vi "FlexRIOonlyResources.vi"() -> ()   [LabVIEW 2013]
uses:
  Control 1.ctl
  ctl.ctl
  <vilib>/Platform/TimedLoop/XDataNode/timing_clust.ctl
  <vilib>/Platform/TimedLoop/XDataNode/nitl_modes.ctl
  <vilib>/Platform/TimedLoop/XDataNode/wakeup.ctl
  Libraries/StateControl.ctl
  Libraries/FlexRIO-NoModule/N Channels.ctl
  <vilib>/rvi/Emulation/niFpgaSctlEmulationGetInTimedLoop.vi
  <vilib>/rvi/Emulation/niFpgaEmulationReportErrorSimple.vi
  <vilib>/rvi/Emulation/niFpgaGetClockAttributes.vi
  <vilib>/rvi/Emulation/niFpgaCriticalErrorInLSC.vi
  <vilib>/rvi/FIFO/Fifo_Resource/nirvififoEmulationClearFpgaImpl.vi
  <vilib>/rvi/DataTransferAndStorage/Container/Common/niFpgaContainerGetUniqueNameForEmu.vi
  Libraries/GlobalReg.vi
  <vilib>/rvi/DataTransferAndStorage/Container/Common/niFpgaContainerExecOnDevCompGetState.vi
  <vilib>/rvi/FIFO/Fifo_Resource/nirvififoEmulationGetNumberOfElementsToReadFpgaImpl.vi
  <vilib>/rvi/interface/RandomDataEmulation/nirviRandomDataFPGAFIFO.vi
  <vilib>/rvi/interface/RandomDataEmulation/niFpgaRandomDataHandleErrors.vi
  <vilib>/rvi/eio/common/nirviEmuReportErrorAndStop.vi
  <vilib>/rvi/FIFO/Fifo_Resource/nirvififoEmulationReadFpgaImpl.vi
  <vilib>/rvi/FIFO/Fifo_Resource/nirvififoEmulationWriteFpgaImpl.vi
  <vilib>/rvi/Emulation/niFpgaProcessEmulError.vi
  <vilib>/rvi/eio/common/nirviEmuTemplateMethod_errors.vi
  <vilib>/Platform/TimedLoop/XDataNode/XDataNode.xnode
  <vilib>/rvi/DataTransferAndStorage/Container/XNode/niFpgaContainer.xnode
  <vilib>/rvi/FIFO/Fifo_Resource/nirvififoEmulationClear.vi
  <vilib>/rvi/FIFO/Fifo_Resource/niFpgaFifoEmulationRefIn.vi
  <vilib>/rvi/interface/RandomDataEmulation/nirviRandomDataFpgaReadWriteTemplate.vi
  <vilib>/eio/EIONode/EIONode.xnode
  <vilib>/Platform/TimedLoop/XDataNode/XDNodeRunTimeDep.lvlib
panel:
  in  "Cluster in":T1
  in  "Tab Control":T2(tab)=enum."Data Acquisition"
  out "Platform":enum8{"FlexRIO", "cRIO", "RSeries"}(ring)
  out "FPGAVIversion":u8[](array[numeric])=[1, 1]
  out "InitDone":bool
  out "RIOAdapterCorrect":bool
  out "Fref":u32=100000000
  out "DevQualityStatus":u8
  out "DevTemp":i16=-10244
  out "DevProfile":u8 format="%x"
  in  "DAQStartStop":bool
  in  "DebugMode":bool
  out "Expected IO Module ID":u32 format="%x"
  out "InsertedIOModule ID":u32
  out "DMATtoHOSTNCh":T3[](array[typedef])=[4]
  out "DMATtoHOSTFrameType":u8[](array[numeric])
  out "DMATtoHOSTSampleSize":u8[](array[numeric])=[2]
  out "DMATtoHOSTBlockNWords":u16[](array[numeric])=[4096]
  in  "DMATtoHOSTSamplingRate0":u16=10000
  in  "DMATtoHOSTEnable0":bool
  out "DMATtoHOSTOverflows":u16
  out "auxAI5":i32
  out "auxAI4":i32
  out "auxAI3":i32
  out "auxAI2":i32
  out "auxAI1":i32
  out "auxAI0":i32
  in  "auxAO5":i32
  in  "auxAO4":i32
  in  "auxAO3":i32
  in  "auxAO2":i32
  in  "auxAO1":i32
  in  "auxAO0":i32
  out "auxDI5":bool
  out "auxDI4":bool
  out "auxDI3":bool
  out "auxDI2":bool
  out "auxDI1":bool
  out "auxDI0":bool
  in  "auxDO3":bool
  in  "auxDO4":bool
  in  "auxDO5":bool
  in  "auxDO2":bool
  in  "auxDO1":bool
  in  "auxDO0":bool
  in  "AOEnable0":bool
  in  "SGUpdateRate0":u32=40
  in  "SGSignalType0":u8
  in  "SGPhase0":u32
  in  "SGFreq0":u32=100000
  in  "SGAmp0":u16
  in  "AO0":i32
  out "SGNo":u8=2 format="%x"
  out "SGFref0":u32=100000000
  out "auxDI6":bool
  out "auxDI7":bool
  out "auxDI8":bool
  out "auxDI9":bool
  out "auxDI10":bool
  out "auxDI11":bool
  out "auxDI12":bool
  out "auxDI13":bool
  out "auxDI14":bool
  out "auxDI15":bool
  in  "auxDO6":bool
  in  "auxDO7":bool
  in  "auxDO8":bool
  in  "auxDO12":bool
  in  "auxDO13":bool
  in  "auxDO14":bool
  in  "auxDO11":bool
  in  "auxDO10":bool
  in  "auxDO9":bool
  in  "auxDO15":bool
  in  "auxAO6":i32
  in  "auxAO7":i32
  in  "auxAO8":i32
  in  "auxAO9":i32
  in  "auxAO10":i32
  in  "auxAO11":i32
  in  "auxAO12":i32
  in  "auxAO13":i32
  in  "auxAO14":i32
  in  "auxAO15":i32
  out "auxAI6":i32
  out "auxAI7":i32
  out "auxAI8":i32
  out "auxAI9":i32
  out "auxAI10":i32
  out "auxAI11":i32
  out "auxAI12":i32
  out "auxAI13":i32
  out "auxAI14":i32
  out "auxAI15":i32
  in  "AOEnable1":bool
  in  "AO1":i32
  in  "SGUpdateRate1":u32=40
  in  "SGFreq1":u32=100000
  out "SGFref1":u32=100000000
  in  "SGPhase1":u32
  in  "SGAmp1":u16
  in  "SGSignalType1":u8
  in  "DO15":bool
  in  "DO14":bool
  in  "DO13":bool
  in  "DO12":bool
  in  "DO9":bool
  in  "DO10":bool
  in  "DO11":bool
  in  "DO8":bool
  in  "DO7":bool
  in  "DO6":bool
  in  "DO3":bool
  in  "DO4":bool
  in  "DO5":bool
  in  "DO2":bool
  in  "DO1":bool
  in  "DO0":bool
  in  "DO18":bool
  in  "DO19":bool
  in  "DO20":bool
  in  "DO17":bool
  in  "DO16":bool
  in  "DO21":bool
  in  "DO24":bool
  in  "DO25":bool
  in  "DO26":bool
  in  "DO23":bool
  in  "DO22":bool
  in  "DO27":bool
  in  "DO30":bool
  in  "DO31":bool
  in  "DO32":bool
  in  "DO33":bool
  in  "DO36":bool
  in  "DO37":bool
  in  "DO38":bool
  in  "DO29":bool
  in  "DO28":bool
  in  "DO39":bool
  in  "DO42":bool
  in  "DO43":bool
  in  "DO44":bool
  in  "DO35":bool
  in  "DO34":bool
  in  "DO45":bool
  in  "DO48":bool
  in  "DO49":bool
  in  "DO50":bool
  in  "DO51":bool
  in  "DO52":bool
  in  "DO40":bool
  in  "DO41":bool
  in  "DO53":bool
  in  "DO46":bool
  in  "DO47":bool
  out "DI11":bool
  out "DI10":bool
  out "DI9":bool
  out "DI8":bool
  out "DI7":bool
  out "DI6":bool
  out "DI15":bool
  out "DI14":bool
  out "DI13":bool
  out "DI12":bool
  out "DI5":bool
  out "DI4":bool
  out "DI3":bool
  out "DI2":bool
  out "DI1":bool
  out "DI0":bool
  out "DI18":bool
  out "DI19":bool
  out "DI20":bool
  out "DI21":bool
  out "DI22":bool
  out "DI23":bool
  out "DI30":bool
  out "DI31":bool
  out "DI32":bool
  out "DI33":bool
  out "DI24":bool
  out "DI25":bool
  out "DI26":bool
  out "DI27":bool
  out "DI28":bool
  out "DI29":bool
  out "DI36":bool
  out "DI37":bool
  out "DI38":bool
  out "DI39":bool
  out "DI40":bool
  out "DI41":bool
  out "DI34":bool
  out "DI35":bool
  out "DI16":bool
  out "DI17":bool
  out "DI42":bool
  out "DI43":bool
  out "DI44":bool
  out "DI45":bool
  out "DI46":bool
  out "DI47":bool
  out "DI51":bool
  out "DI52":bool
  out "DI53":bool
  out "DI48":bool
  out "DI49":bool
  out "DI50":bool
  # "Inputs"
  # "Aux Analog Input"
  # "Aux Digital Input"
  # "Digital Inputs"
  # "Outputs"
  # "Analog Outputs"
  # "Number of WF gen"
  # "Digital Outputs"
  # "Signal Generator 0"
  # "Signal Generator 1"
  # "Aux Digital Output"
  # "Aux Analog Output"
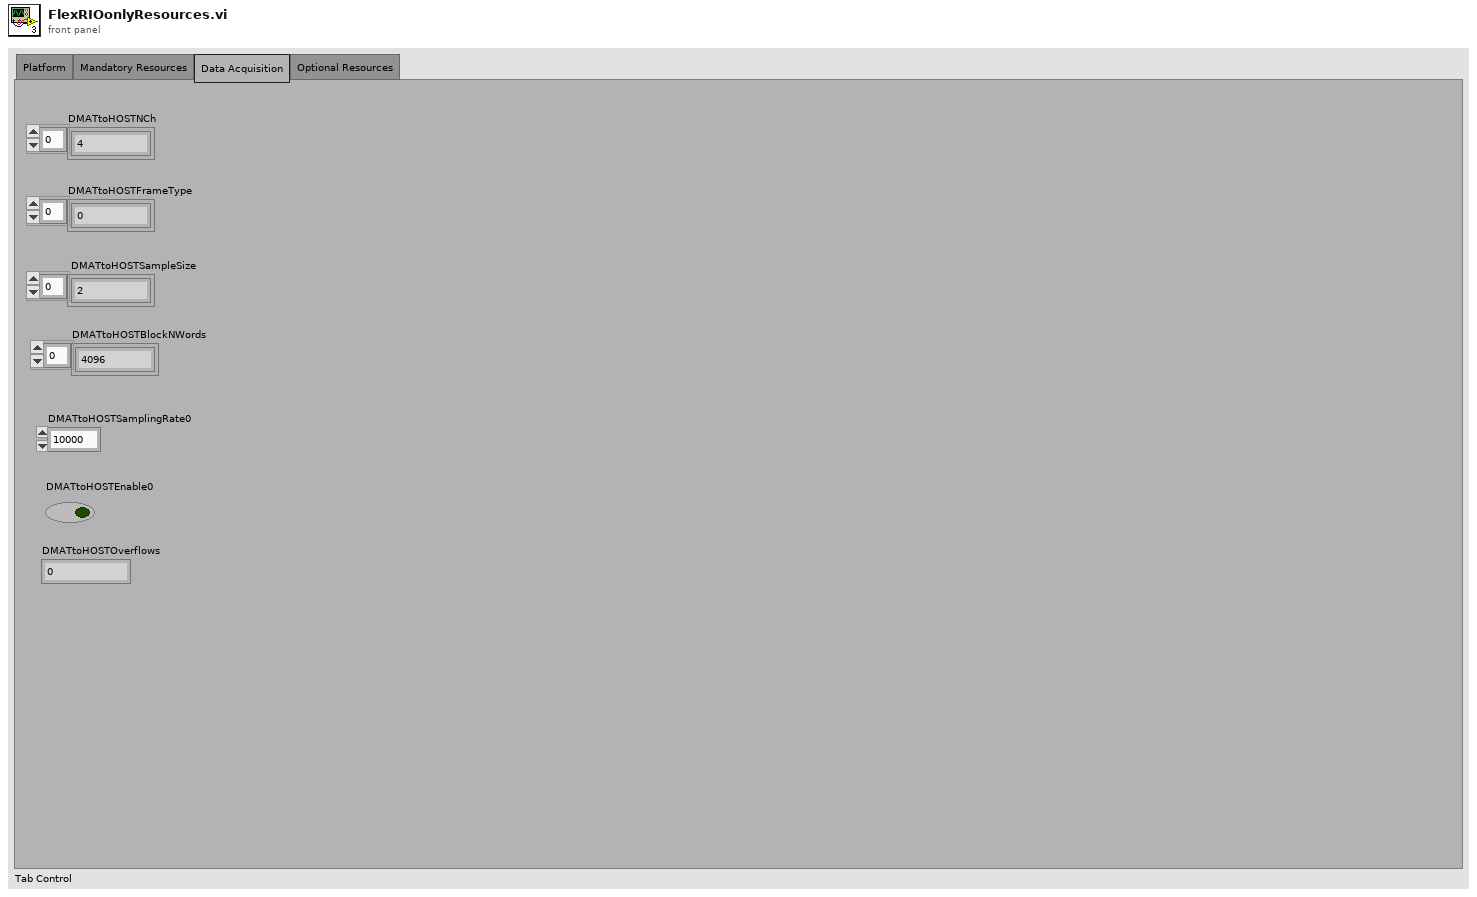
[diagram p1: front panel]
types:
  T1 = typedef "ctl.ctl" = cluster{"Number of sample in a block (0-4095)":u16, "SamplingRateN (Default 5000) (Decimation factor from ref clock)":u16, "Channels shif register up to 4 (A) ":u64, "Channels shif register up to 4 (B) ":u64, "Channels shif register up to 4 (C) ":u64, "Info shift register":u64, "ramp counter":i16, "GroupEnableN":bool, "Debug activation":bool, "Sample counter ":u64, "Decimation counter":u16, "Blocks counter":u16}
  T2 = enum32{"Platform", "Mandatory Resources", "Data Acquisition", "Optional Resources"}
  T3 = typedef "Control 1.ctl" = u16
  T4 = typedef "XDNodeRunTimeDep.lvlib/timing_clust.ctl" = cluster{"Expected End [f-1]":u64, "Actual End [f-1]":u64, "Finished Late? [f-1]":bool, "Expected End [i-1]":u64, "Actual End [i-1]":u64, "Finished Late? [i-1]":bool, "Expected Start [i]":u64, "Actual Start [i]":u64, "Expected Start [f]":u64, "Actual Start [f]":u64, "Source Name":string, "Structure Name":string, "Period":i64, "Deadline":i64, "Offset":i64, "Start":i64, "Priority":i32, "Timeout":i32, "Mode":T5, "Wakeup Reason":T6, "Error":errorcluster, "Source Type":string, "Secondary Source Type":string, "Global End Time":u64, "Global Start Time":u64, "Frame Duration":u64, "Iteration Duration":u64, "Assigned CPU":i32, "I/O Scan Engine Mode":u32}
  T5 = typedef "XDNodeRunTimeDep.lvlib/nitl_modes.ctl" = enum32{"No Change", "Process missed periods, maintain original phase", "Discard missed periods, maintain original phase", "Process missed periods, ignore original phase", "Discard missed periods, ignore original phase"}
  T6 = typedef "XDNodeRunTimeDep.lvlib/wakeup.ctl" = enum32{"Normal", "Aborted", "Asynchronous wakeup", "Timing source error", "Timed loop error", "Timeout"}
  T7 = typedef "StateControl.ctl" = enum16{"Idle", "Acq"}
  T8 = typedef "N Channels.ctl" = enum16{"0 Channels", "1 Channels", "2 Channels", "3 Channels", "4 Channels", "5 Channels", "6 Channels", "7 Channels", "8 Channels", "9 Channels", "10 Channels", "11 Channels", "12 Channels"}
  T9 = cluster{u16, u16, u64, u64, u64, u64, i16, bool, bool, u64, u16, u16}
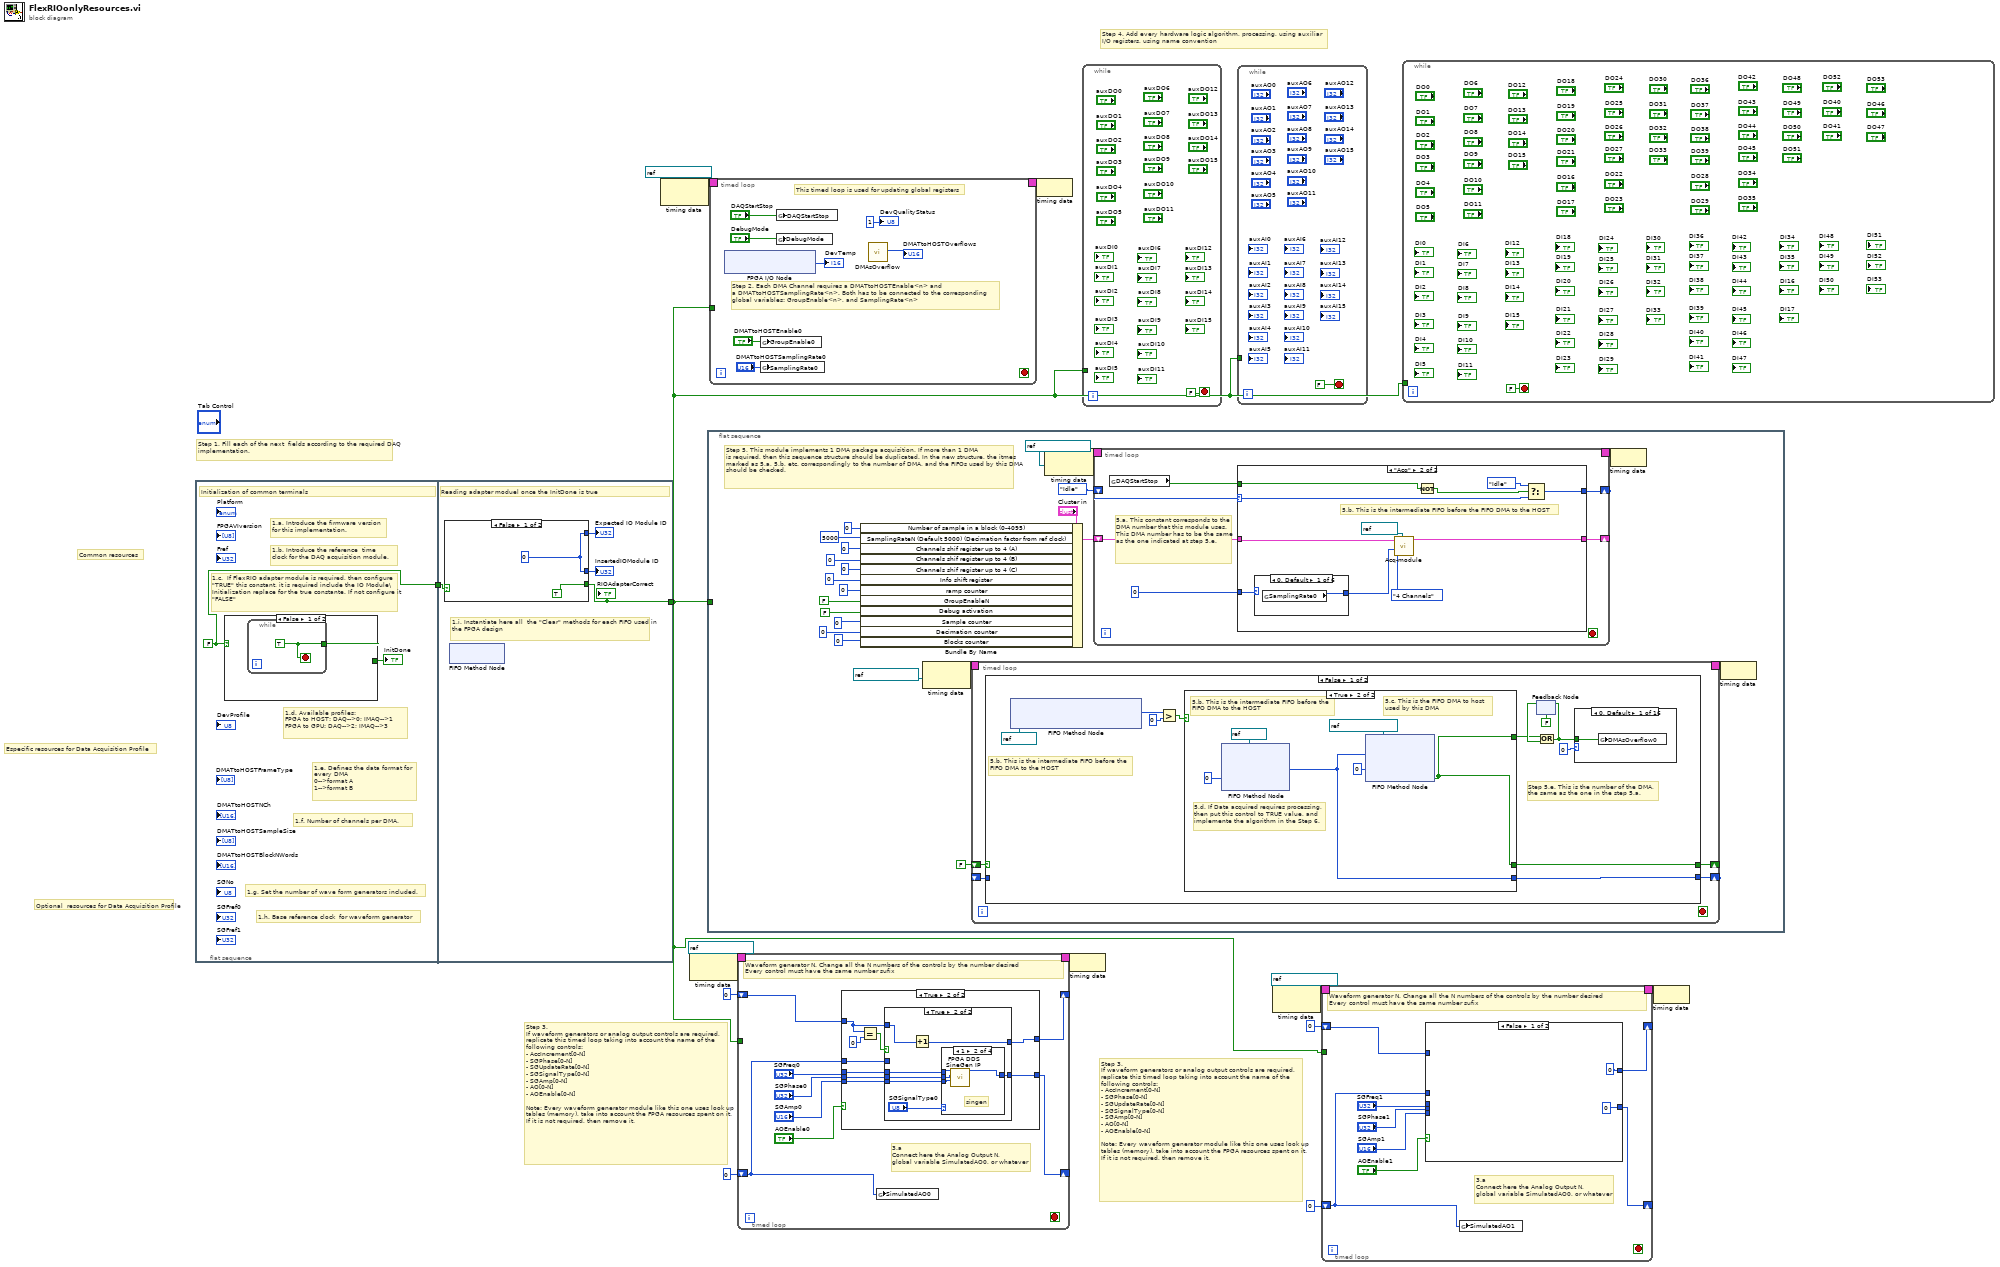
[diagram p0: block diagram]
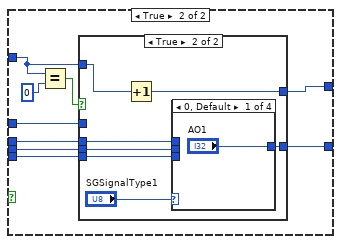
[diagram p2: hidden frame]
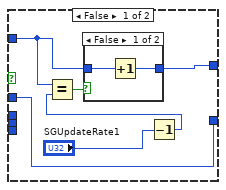
[diagram p3: hidden frame]
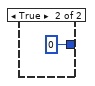
[diagram p4: hidden frame]
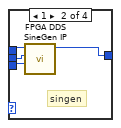
[diagram p5: hidden frame]
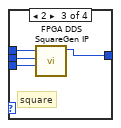
[diagram p6: hidden frame]
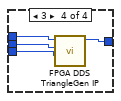
[diagram p7: hidden frame]
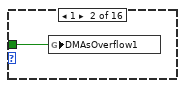
[diagram p8: hidden frame]
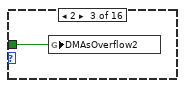
[diagram p9: hidden frame]
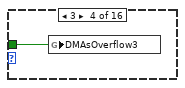
[diagram p10: hidden frame]
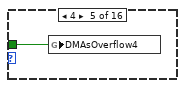
[diagram p11: hidden frame]
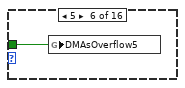
[diagram p12: hidden frame]
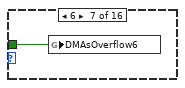
[diagram p13: hidden frame]
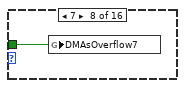
[diagram p14: hidden frame]
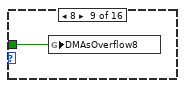
[diagram p15: hidden frame]
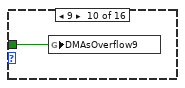
[diagram p16: hidden frame]
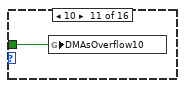
[diagram p17: hidden frame]
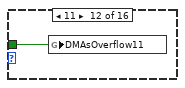
[diagram p18: hidden frame]
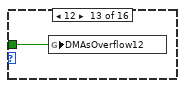
[diagram p19: hidden frame]
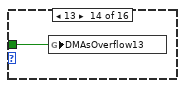
[diagram p20: hidden frame]
diagram:
  # "Step 3.\nIf waveform generators or analog output controls are required,\nreplicate this timed loop taking into account the name of the \nfollowing controls:\n- AccIncrement[0-N]\n- SGPhase[0-N]\n- SGUpdateRate[0-N]\n- SGSignalType[0-N]\n- SGAmp[0-N]\n- AO[0-N]\n- AOEnable[0-N]\n\nNote: Every waveform generator module like this one uses look up tables (memory), take into account the FPGA resources spent on it.  If it is not required, then remove it."
  # "Optional  resources for Data Acquisition Profile"
  # "Especific resources for Data Acquisition Profile"
  # "Common resources"
  # "Step 4. Add every hardware logic algorithm, processing, using auxiliar \nI/O registers, using name convention"
  # "Step 3.\nIf waveform generators or analog output controls are required,\nreplicate this timed loop taking into account the name of the \nfollowing controls:\n- AccIncrement[0-N]\n- SGPhase[0-N]\n- SGUpdateRate[0-N]\n- SGSignalType[0-N]\n- SGAmp[0-N]\n- AO[0-N]\n- AOEnable[0-N]\n\nNote: Every waveform generator module like this one uses look up tables (memory), take into account the FPGA resources spent on it.  If it is not required, then remove it."
  # "Step 1. Fill each of the next  fields according to the required DAQ implementation."
  n1 = flat-sequence {
    tunnel: [w16] -> w15
    tunnel: [w23] -> w1
    tunnel: w15 -> [w22]
    frame #0 {
      w16 = FALSE
      # "1.h. Base reference clock  for waveform generator"
      # "1.e. Defines the data format for \nevery DMA\n0-->format A\n1-->format B"
      # "1.c.  If FlexRIO adapter module is required, then configure \"TRUE\" this constant, it is required include the IO Module\\Initialization replace for the true constante. If not configure it \"FALSE\""
      # "1.a. Introduce the firmware version \nfor this implementation."
      # "1.b. Introduce the reference  time \nclock for the DAQ acquisition module."
      # "1.g. Set the number of wave form generators included."
      # "1.f. Number of channels per DMA."
      # "1.d. Available profiles: \nFPGA to HOST: DAQ-->0; IMAQ-->1\nFPGA to GPU: DAQ-->2; IMAQ-->3"
      # "Initialization of common terminals"
      n2 = case shown="False" w16 {
        tunnel: [w18 w20] -> w17
        frame False {
          n3 = while {
            tunnel: [w19] -> w18
            stop <- w19 stop-if-true
            w19 = TRUE
          }
        }
        frame True {
          n4 = while {
            tunnel: [w21] -> w20
            stop <- w21 stop-if-true
            w21 = TRUE
          }
        }
      }
      "InitDone" <- w17
    }
    frame #1 {
      # "1.i. Instantiate here all  the \"Clear\" methods for each FIFO used in the FPGA design"
      # "Reading adapter moduel once the InitDone is true"
      n5 = case shown="False" w22 {
        tunnel: [TRUE w30] -> w23
        tunnel: [w27 w29] -> w25
        tunnel: [w27 w28] -> w24
        frame False {
          w27 = u32 0
        }
        frame True {
          n6 = xnode "FPGA I/O Node"() -> ("Expected IO Module ID"=w29:u32)  [unwired: 1 in, 1 out]
          n7 = xnode "FPGA I/O Node"() -> ("Inserted IO Module ID"=w28:u32)  [unwired: 1 in, 1 out]
          n8 = Equal?(x=w29, y=w28) -> (x = y?=w30:bool)
        }
      }
      "Expected IO Module ID" <- w25
      "InsertedIOModule ID" <- w24
      "RIOAdapterCorrect" <- w23
      n9 = xnode ("FIFO Method Node")() -> ()  [unwired: 1 in, 1 out]
    }
  }
  n10 = node-c288(refnum<k21> "100 MHz Clock" ("Source Name")) -> (w9:T4)
  n11 = node-c288(refnum<k21> "100 MHz Clock" ("Source Name")) -> (w14:T4)
  n12 = flat-sequence {
    tunnel: w1 -> [_]
    frame #0 {
      # "Step 5. This module implements 1 DMA package acquisition. If more than 1 DMA \nis required, then this sequence structure should be duplicated. In the new structure, the itmes marked as 5.a, 5.b, etc. correspondingly to the number of DMA, and the FIFOs used by this DMA should be checked."
      n13 = Bundle By Name(cluster="Cluster in", "Number of sample in a block (0-4095)"=u16 0 ("sample of block out"), "SamplingRateN (Default 5000) (Decimation factor from ref clock)"=u16 5000 ("FS1"), "Channels shif register up to 4 (A)"=u64 0, "Channels shif register up to 4 (B)"=u64 0, "Channels shif register up to 4 (C)"=u64 0, "Info shift register"=u64 0 ("Element"), "ramp counter"=i16 0, "GroupEnableN"=FALSE ("DMA1activation"), "Debug activation"=FALSE, "Sample counter"=u64 0 ("contador muestra"), "Decimation counter"=u16 0, "Blocks counter"=u16 0) -> (w33:T1)
      n14 = node-c288(refnum<k21> "100 MHz Clock" ("Source Name")) -> (w50:T4)
      n15 = timed-loop {
        timing: w50 -> [_]
        timing-out: [_] -> w49
        shift-right: [w56] -> _
        shift-left: FALSE ("Timed Out?") -> [w55]
        shift-right: [w54] -> _
        shift-left: _ -> [w53]
        stop <- _ stop-if-true
        n16 = case shown="False" w55 {
          tunnel: [w61 w93] -> w56
          tunnel: [w60 w92] -> w54
          tunnel: w53 -> [_ w92]
          frame False {
            # "Step 5.e. This is the number of the DMA,\nthe same as the one in the step 5.a."
            # "5.b. This is the intermediate FIFO before the \nFIFO DMA to the HOST"
            n17 = xnode ("FIFO Method Node")("FIFO In"=refnum<k21> "FIFO0" ("IntermediateFIFO")) -> ("Number of Elements to Read"=w64:u32)  [unwired: 1 out]
            n18 = Greater?(x=w64, y=u32 0) -> (0:w62:bool)
            n19 = case shown="True" w62 {
              tunnel: [FALSE ("Timed Out?") w89] -> w65
              tunnel: [FALSE ("Timed Out?") w89] -> w61
              tunnel: [_ w88] -> w60
              frame False {
              }
              frame True {
                # "5.d. If Data acquired requires processing,\nthen put this control to TRUE value, and\nimplemente the algorithm in the Step 6."
                # "5.c. This is the FIFO DMA to host \nused by this DMA"
                # "5.b. This is the intermediate FIFO before the \nFIFO DMA to the HOST"
                n20 = xnode ("FIFO Method Node")("Timeout"=0, "FIFO In"=refnum<k21> "FIFO0" ("IntermediateFIFO")) -> ("Element"=w88:u64)  [unwired: 2 out]
                n21 = xnode ("FIFO Method Node")("Element"=w88, "Timeout"=0, "FIFO In"=refnum<k21> "DMATtoHOST0") -> ("Timed Out?"=w89:bool)  [unwired: 1 out]
              }
            }
            n22 = feedback #1(FALSE) -> (w66:bool)
            n23 = Or(x=w65, y=w66) -> (x .or. y?=w59:bool)
            n24 = feedback-in #1(w59) -> ()
            n25 = case shown="0, Default" i16 0 ("DMA number") {
              tunnel: w59 -> [w68 w69 w70 w71 w72 w73 w74 w75 w76 w77 w78 w79 w80 w81 w82 w83]
              frame 0, Default {
                n26 = global write "GlobalReg.vi" "DMAsOverflow0"(w68) -> ()
              }
              frame 1 {
                n27 = global write "GlobalReg.vi" "DMAsOverflow1"(w69) -> ()
              }
              frame 2 {
                n28 = global write "GlobalReg.vi" "DMAsOverflow2"(w70) -> ()
              }
              frame 3 {
                n29 = global write "GlobalReg.vi" "DMAsOverflow3"(w71) -> ()
              }
              frame 4 {
                n30 = global write "GlobalReg.vi" "DMAsOverflow4"(w72) -> ()
              }
              frame 5 {
                n31 = global write "GlobalReg.vi" "DMAsOverflow5"(w73) -> ()
              }
              frame 6 {
                n32 = global write "GlobalReg.vi" "DMAsOverflow6"(w74) -> ()
              }
              frame 7 {
                n33 = global write "GlobalReg.vi" "DMAsOverflow7"(w75) -> ()
              }
              frame 8 {
                n34 = global write "GlobalReg.vi" "DMAsOverflow8"(w76) -> ()
              }
              frame 9 {
                n35 = global write "GlobalReg.vi" "DMAsOverflow9"(w77) -> ()
              }
              frame 10 {
                n36 = global write "GlobalReg.vi" "DMAsOverflow10"(w78) -> ()
              }
              frame 11 {
                n37 = global write "GlobalReg.vi" "DMAsOverflow11"(w79) -> ()
              }
              frame 12 {
                n38 = global write "GlobalReg.vi" "DMAsOverflow12"(w80) -> ()
              }
              frame 13 {
                n39 = global write "GlobalReg.vi" "DMAsOverflow13"(w81) -> ()
              }
              frame 14 {
                n40 = global write "GlobalReg.vi" "DMAsOverflow14"(w82) -> ()
              }
              frame 15 {
                n41 = global write "GlobalReg.vi" "DMAsOverflow15"(w83) -> ()
              }
            }
          }
          frame True {
            n42 = xnode ("FIFO Method Node")("Element"=w92, "Timeout"=0) -> ("Timed Out?"=w93:bool)  [unwired: 1 in, 1 out]
          }
        }
      }
      n43 = node-c288(refnum<k21> "100 MHz Clock" ("Source Name")) -> (w52:T4)
      n44 = timed-loop {
        timing: w52 -> [_]
        timing-out: [_] -> w51
        shift-right: [w105] -> _
        shift-left: StateControl."Idle" ("Enum") -> [w106]
        shift-right: [w102] -> _
        shift-left: w33 -> [w103]
        stop <- _ stop-if-true
        # "5.a. This constant corresponds to the DMA number that this module uses. This DMA number has to be the same as the one indicated at step 5.e."
        n45 = global read "GlobalReg.vi" "DAQStartStop"() -> (w104:bool)
        n46 = case shown="\"Acq\"" w106 {
          selector: w106 -> [w116 w134]
          tunnel: w104 -> [w118 w125]
          tunnel: [w115 w133] -> w105
          tunnel: w103 -> [w114 w131]
          tunnel: [w109 w130] -> w102
          tunnel: i16 0 ("DMA number") -> [w107 w127]
          frame "Idle", Default {
            w108 = i16 0
            n47 = case shown="0, Default" w107 {
              tunnel: [w119 w120 w121 w122 w123 w124] -> w110
              frame 0, Default {
                n48 = global read "GlobalReg.vi" "GroupEnable0"() -> (w119:bool)
              }
              frame 1 {
                n49 = global read "GlobalReg.vi" "GroupEnable1"() -> (w120:bool)
              }
              frame 2 {
                n50 = global read "GlobalReg.vi" "GroupEnable2"() -> (w121:bool)
              }
              frame 3 {
                n51 = global read "GlobalReg.vi" "GroupEnable3"() -> (w122:bool)
              }
              frame 4 {
                n52 = global read "GlobalReg.vi" "GroupEnable4"() -> (w123:bool)
              }
              frame 5 {
                n53 = global read "GlobalReg.vi" "GroupEnable5"() -> (w124:bool)
              }
            }
            n54 = global read "GlobalReg.vi" "DebugMode"() -> (w111:bool)
            n55 = Bundle By Name(cluster=w114, "Number of sample in a block (0-4095)"=u16 0, "ramp counter"=u64 0, "GroupEnableN"=w110, "Debug activation"=w111, "Sample counter"=w108, "Decimation counter"=w108, "Blocks counter"=w108) -> (w109:T1)
            n56 = Select(t=StateControl."Acq" ("Enum"), s=w118, f=w116) -> (s? t:f=w115:T7)
          }
          frame "Acq" {
            # "5.b. This is the intermediate FIFO before the FIFO DMA to the HOST"
            n57 = case shown="0, Default" w127 {
              tunnel: [w136 w137 w138 w139 w140 w141] -> w132
              frame 0, Default {
                n58 = global read "GlobalReg.vi" "SamplingRate0"() -> (w136:u16)
              }
              frame 1 {
                n59 = global read "GlobalReg.vi" "SamplingRate1"() -> (w137:u16)
              }
              frame 2 {
                n60 = global read "GlobalReg.vi" "SamplingRate2"() -> (w138:u16)
              }
              frame 3 {
                n61 = global read "GlobalReg.vi" "SamplingRate3"() -> (w139:u16)
              }
              frame 4 {
                n62 = global read "GlobalReg.vi" "SamplingRate4"() -> (w140:u16)
              }
              frame 5 {
                n63 = global read "GlobalReg.vi" "SamplingRate5"() -> (w141:u16)
              }
            }
            n64 = call "Acq-module.vi"("IntermediateFIFO"=refnum<k21> "FIFO0", "NumChannels"=N_Channels."4 Channels", "SamplingRate0"=w132, "Cluster in"=w131) -> ("cluster out"=w130:T9)  [unwired: 7 in]
            n65 = Not(x=w125) -> (.not. x?=w126:bool)
            n66 = Select(t=StateControl."Idle" ("Enum"), s=w126, f=w134) -> (s? t:f=w133:T7)
          }
        }
      }
      n67 = node-c288(w51) -> ()
      n68 = node-c288(w49) -> ()
    }
  }
  n69 = timed-loop {
    timing: w9 -> [_]
    timing-out: [_] -> w8
    tunnel: w1 -> [_]
    stop <- _ stop-if-true
    # "This timed loop is used for updating global registers"
    # "Step 2. Each DMA Channel requires a DMATtoHOSTEnable<n> and\na DMATtoHOSTSamplingRate<n>. Both has to be connected to the corresponding\nglobal variables: GroupEnable<n>, and SamplingRate<n>"
    n70 = xnode "FPGA I/O Node"() -> ("Device Temperature"=→"DevTemp":i16)  [unwired: 1 in, 1 out]
    n71 = global write "GlobalReg.vi" "GroupEnable0"("DMATtoHOSTEnable0") -> ()
    n72 = global write "GlobalReg.vi" "SamplingRate0"("DMATtoHOSTSamplingRate0") -> ()
    n73 = global write "GlobalReg.vi" "DebugMode"("DebugMode") -> ()
    n74 = global write "GlobalReg.vi" "DAQStartStop"("DAQStartStop") -> ()
    n75 = call "DMAsOverflow.vi"() -> ("DMAsOverFlow"=→"DMATtoHOSTOverflows":u16)  [unwired: 11 in]
    "DevQualityStatus" <- u8 1 ("DevQualityStatus")
  }
  n76 = timed-loop {
    shift-right: [w160] -> _
    shift-left: i16 0 ("Signal Value") -> [w157]
    timing: w14 -> [_]
    timing-out: [_] -> w13
    shift-right: [w158] -> _
    shift-left: u32 0 -> [w159]
    tunnel: w1 -> [_]
    stop <- _ stop-if-true
    # "3.a\nConnect here the Analog Output N,\nglobal variable SimulatedAO0, or whatever"
    # "Waveform generator N. Change all the N numbers of the controls by the number desired\nEvery control must have the same number sufix"
    n77 = case shown="True" "AOEnable0" {
      tunnel: "SGFreq0" -> [_ w175]
      tunnel: "SGPhase0" -> [_ w174]
      tunnel: "SGAmp0" -> [_ w173]
      tunnel: [i16 0 w172] -> w160
      tunnel: w159 -> [_ w169]
      tunnel: [u32 0 w168] -> w158
      tunnel: w157 -> [_ w167]
      frame False {
      }
      frame True {
        n78 = Equal?(x=w169, y=u32 0) -> (x = y?=w171:bool)
        n79 = case shown="True" w171 {
          tunnel: w175 -> [_ w191]
          tunnel: w174 -> [_ w190]
          tunnel: w173 -> [_ w189]
          tunnel: [w180 w188] -> w172
          tunnel: w169 -> [w179 w186]
          tunnel: [w181 w185] -> w168
          tunnel: w167 -> [w180 _]
          frame False {
            n80 = Decrement(x="SGUpdateRate0") -> (x-1=w177:u32)
            n81 = Equal?(x=w179, y=w177) -> (x = y?=w178:bool)
            n82 = case shown="False" w178 {
              tunnel: w179 -> [w183 _]
              tunnel: [w182 u32 0] -> w181
              frame False {
                n83 = Increment(x=w183) -> (x+1=w182:u32)
              }
              frame True {
              }
            }
          }
          frame True {
            n84 = Increment(x=w186) -> (x+1=w185:u32)
            n85 = case shown="1" "SGSignalType0" {
              tunnel: w191 -> [_ w196 w200 w204]
              tunnel: w190 -> [_ w195 w199 w203]
              tunnel: w189 -> [_ w194 w198 w202]
              tunnel: ["AO0" w193 w197 w201] -> w188
              frame 0, Default {
              }
              frame 1 {
                # "singen"
                n86 = call "FPGA DDS SineGen IP.vi"("Signal Amplitude (x 2^15)"=w194, "Phase Shift"=w195, "Accumulator Increment"=w196) -> ("Signal Value"=w193:i16)  [unwired: 7 in, 1 out]
              }
              frame 2 {
                # "square"
                n87 = call "FPGA DDS SquareGen IP.vi"("Signal Amplitude (x 2^15)"=w198, "Phase Shift"=w199, "Accumulator Increment"=w200) -> ("Signal Value"=w197:i16)  [unwired: 7 in, 1 out]
              }
              frame 3 {
                n88 = call "FPGA DDS TriangleGen IP.vi"("Signal Amplitude (x 2^15)"=w202, "Phase Shift"=w203, "Accumulator Increment"=w204) -> ("Signal Value"=w201:i16)  [unwired: 7 in, 1 out]
              }
            }
          }
        }
      }
    }
    n89 = global write "GlobalReg.vi" "SimulatedAO0"(w157) -> ()
  }
  n90 = node-c288(w8) -> ()
  n91 = node-c288(w13) -> ()
  n92 = while {
    tunnel: w1 -> [_]
    stop <- FALSE stop-if-true
  }
  n93 = while {
    tunnel: w1 -> [_]
    stop <- FALSE stop-if-true
  }
  n94 = node-c288(refnum<k21> "100 MHz Clock" ("Source Name")) -> (w6:T4)
  n95 = timed-loop {
    shift-right: [w212] -> _
    shift-left: i16 0 ("Signal Value") -> [w209]
    timing: w6 -> [_]
    timing-out: [_] -> w5
    shift-right: [w210] -> _
    shift-left: u32 0 -> [w211]
    tunnel: w1 -> [_]
    stop <- _ stop-if-true
    # "3.a\nConnect here the Analog Output N,\nglobal variable SimulatedAO0, or whatever"
    # "Waveform generator N. Change all the N numbers of the controls by the number desired\nEvery control must have the same number sufix"
    n96 = case shown="False" "AOEnable1" {
      tunnel: "SGFreq1" -> [_ w227]
      tunnel: "SGPhase1" -> [_ w226]
      tunnel: "SGAmp1" -> [_ w225]
      tunnel: [i16 0 w224] -> w212
      tunnel: w211 -> [_ w221]
      tunnel: [u32 0 w220] -> w210
      tunnel: w209 -> [_ w219]
      frame False {
      }
      frame True {
        n97 = Equal?(x=w221, y=u32 0) -> (x = y?=w223:bool)
        n98 = case shown="True" w223 {
          tunnel: w227 -> [_ w243]
          tunnel: w226 -> [_ w242]
          tunnel: w225 -> [_ w241]
          tunnel: [w232 w240] -> w224
          tunnel: w221 -> [w231 w238]
          tunnel: [w233 w237] -> w220
          tunnel: w219 -> [w232 _]
          frame False {
            n99 = Decrement(x="SGUpdateRate1") -> (x-1=w229:u32)
            n100 = Equal?(x=w231, y=w229) -> (x = y?=w230:bool)
            n101 = case shown="False" w230 {
              tunnel: w231 -> [w235 _]
              tunnel: [w234 u32 0] -> w233
              frame False {
                n102 = Increment(x=w235) -> (x+1=w234:u32)
              }
              frame True {
              }
            }
          }
          frame True {
            n103 = Increment(x=w238) -> (x+1=w237:u32)
            n104 = case shown="0, Default" "SGSignalType1" {
              tunnel: w243 -> [_ w248 w252 w256]
              tunnel: w242 -> [_ w247 w251 w255]
              tunnel: w241 -> [_ w246 w250 w254]
              tunnel: ["AO1" w245 w249 w253] -> w240
              frame 0, Default {
              }
              frame 1 {
                # "singen"
                n105 = call "FPGA DDS SineGen IP.vi"("Signal Amplitude (x 2^15)"=w246, "Phase Shift"=w247, "Accumulator Increment"=w248) -> ("Signal Value"=w245:i16)  [unwired: 7 in, 1 out]
              }
              frame 2 {
                # "square"
                n106 = call "FPGA DDS SquareGen IP.vi"("Signal Amplitude (x 2^15)"=w250, "Phase Shift"=w251, "Accumulator Increment"=w252) -> ("Signal Value"=w249:i16)  [unwired: 7 in, 1 out]
              }
              frame 3 {
                n107 = call "FPGA DDS TriangleGen IP.vi"("Signal Amplitude (x 2^15)"=w254, "Phase Shift"=w255, "Accumulator Increment"=w256) -> ("Signal Value"=w253:i16)  [unwired: 7 in, 1 out]
              }
            }
          }
        }
      }
    }
    n108 = global write "GlobalReg.vi" "SimulatedAO1"(w209) -> ()
  }
  n109 = while {
    tunnel: w1 -> [_]
    stop <- FALSE stop-if-true
  }
  n110 = node-c288(w5) -> ()
